vi "LinuxFreeMem.vi"(8 "error in":errorcluster) -> (0 "error out":errorcluster, 3 "FreeMem":u32)   [LabVIEW 2018]
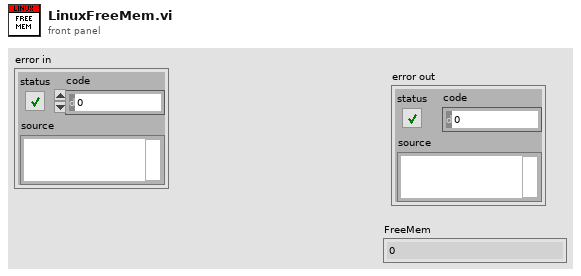
[diagram p1: front panel]
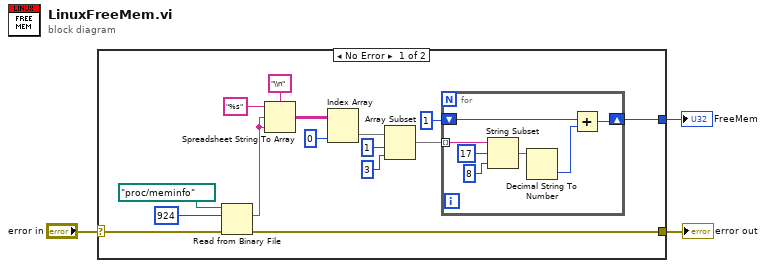
[diagram p0: block diagram]
diagram:
  n1 = case shown="No Error" "error in" {
    selector: "error in" -> [w4 w26]
    tunnel: [w16 w26] -> w3
    tunnel: [w5 _] -> w2
    frame No Error {
      n2 = Read from Binary File(8:w4, 10:924 ("count (1)"), 11:path "/proc/meminfo" ("file (use dialog)")) -> (0:w16:errorcluster, 2:w13:string)  [unwired: 3 in, 2 out]
      n3 = Spreadsheet String To Array(delimiter (Tab)="\\n", format string="%s", spreadsheet string=w13, array type (2D Dbl)=w13) -> (array=w12:string[][])
      n4 = Index Array(array=w12, index (col)=0 ("disabled index (col)")) -> (element=w8:string[])  [unwired: 1 in]
      n5 = Array Subset(array=w8, index=1, length=3) -> (w7:string[])
      n6 = for {
        tunnel: w7 -> [w25] mode=indexing
        shift-right: [w20] -> w5
        shift-left: u32 1 ("index") -> [w21]
        n7 = String Subset(string=w25, offset (0)=17, length (rest)=8 ("length (rest)")) -> (substring=w22:string)
        n8 = Decimal String To Number(string=w22) -> (number=w19:i32)  [unwired: 2 in, 1 out]
        n9 = Add(x=w21, y=w19) -> (x+y=w20:u32)
      }
    }
    frame Error {
    }
  }
  "error out" <- w3
  "FreeMem" <- w2
